vi "MIMIC RecvCommand_safe.vi"(3 "error in":errorcluster, 5 "VISA resource name":refnum<visa-resource-name>) -> (0 "error out":errorcluster, 1 "Receive_buffer":u8[](array[numeric]), 2 "VISA resource name OUT":refnum<visa-resource-name>)   [LabVIEW 2014]
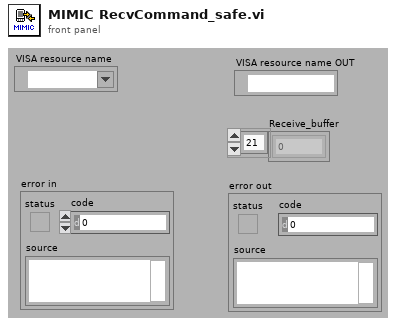
[diagram p1: front panel]
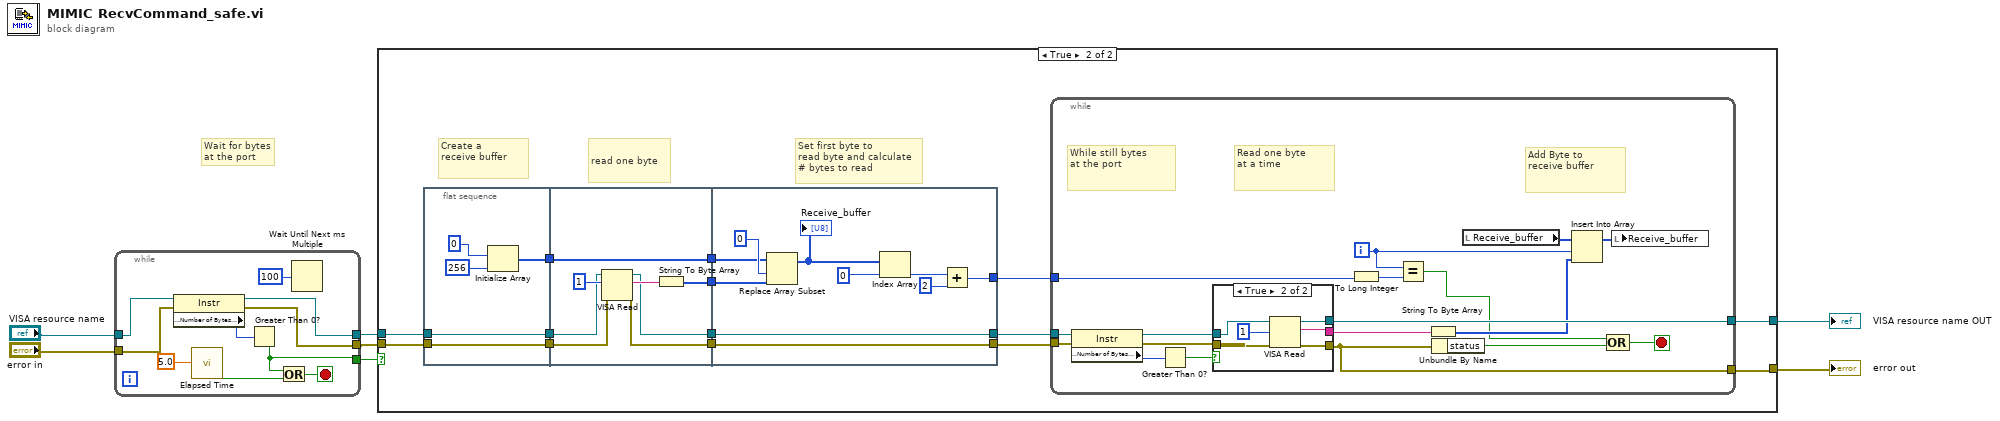
[diagram p0: block diagram]
diagram:
  # "Wait for bytes\nat the port"
  n1 = while {
    tunnel: "error in" -> [w10]
    tunnel: [w14] -> w7
    tunnel: "VISA resource name" -> [w13]
    tunnel: [w12] -> w6
    tunnel: [w8] -> w3
    stop <- w15 stop-if-true
    n2 = property class="Instr"(reference=w13, error in=w10) -> (reference out=w12:refnum<visa-resource-name>, error out=w14:errorcluster, "Serial Settings:Number of Bytes at Serial Port"=w17:u32)
    n3 = call "Elapsed Time"("Time Target (s)"=5.0) -> ("Time has Elapsed"=w16:bool)  [unwired: 11 in, 7 out]
    n4 = Greater Than 0?(x=w17) -> (x > 0?=w8:bool)
    n5 = Or(x=w8, y=w16) -> (x .or. y?=w15:bool)
    n6 = Wait Until Next ms Multiple(millisecond multiple=u32 100) -> ()  [unwired: 1 out]
  }
  n7 = case shown="True" w3 {
    tunnel: w7 -> [w18 w21]
    tunnel: w6 -> [w19 w22]
    tunnel: [w19 w33] -> w1
    tunnel: [w18 w32] -> w2
    frame False {
      # "No Bytes at the port, and we timed out"
    }
    frame True {
      # "Set first byte to \nread byte and calculate # bytes to read"
      # "read one byte"
      # "Create a\nreceive buffer"
      n8 = flat-sequence {
        tunnel: w22 -> [w37]
        tunnel: w21 -> [w38]
        tunnel: [w34] -> w25
        tunnel: [w38] -> w24
        tunnel: [w37] -> w23
        tunnel: [w39] -> w30
        tunnel: [w40] -> w29
        tunnel: [w42] -> w27
        tunnel: w25 -> [w39]
        tunnel: w24 -> [w41]
        tunnel: w23 -> [w43]
        tunnel: [w44] -> w20
        tunnel: [w52] -> w31
        tunnel: w30 -> [w47]
        tunnel: w29 -> [w50]
        tunnel: [w50] -> w28
        tunnel: w27 -> [w49]
        tunnel: [w49] -> w26
        tunnel: w20 -> [w48]
        frame #0 {
          n9 = Initialize Array(u8 0 ("element"), 256 ("dimension size")) -> (w34:u8[])
        }
        frame #1 {
          n10 = VISA Read(VISA resource name=w43, byte count=u32 1, error in (no error)=w41) -> (VISA resource name out=w42:refnum<visa-resource-name>, read buffer=w46:string, error out=w40:errorcluster)  [unwired: 1 out]
          n11 = String To Byte Array(string=w46) -> (unsigned byte array=w44:u8[])
        }
        frame #2 {
          n12 = Replace Array Subset(array=w47, new element=w48, index=0) -> (w56:u8[])
          "Receive_buffer" <- w56
          n13 = Index Array(array=w56, index=0) -> (element=w55:u8)
          n14 = Add(x=w55, y=u8 2) -> (x+y=w52:u8)
        }
      }
      n15 = while {
        tunnel: w26 -> [w72]
        tunnel: w28 -> [w71]
        tunnel: [w67] -> w33
        tunnel: [w64] -> w32
        tunnel: w31 -> [w61]
        i -> [w57]
        stop <- w68 stop-if-true
        # "Add Byte to \nreceive buffer"
        # "Read one byte\nat a time"
        # "While still bytes\nat the port"
        n16 = property class="Instr"(reference=w72, error in=w71) -> (reference out=w70:refnum<visa-resource-name>, error out=w69:errorcluster, "Serial Settings:Number of Bytes at Serial Port"=w74:u32)
        n17 = Greater Than 0?(x=w74) -> (x > 0?=w73:bool)
        n18 = case shown="True" w73 {
          tunnel: w69 -> [w76 w82]
          tunnel: w70 -> [w75 w81]
          tunnel: [w76 w80] -> w64
          tunnel: [_ w79] -> w66
          tunnel: [w75 w78] -> w67
          frame False {
          }
          frame True {
            n19 = VISA Read(VISA resource name=w81, byte count=u32 1, error in (no error)=w82) -> (VISA resource name out=w78:refnum<visa-resource-name>, read buffer=w79:string, error out=w80:errorcluster)  [unwired: 1 out]
          }
        }
        n20 = To Long Integer(number=w61) -> (32bit integer=w58:i32)
        n21 = Equal?(x=w57, y=w58) -> (x = y?=w60:bool)
        n22 = String To Byte Array(string=w66) -> (unsigned byte array=w65:u8[])
        n23 = Unbundle By Name(w64) -> ("status"=w59:bool)
        n24 = local read "Receive_buffer"() -> (w63:u8[])
        n25 = Insert Into Array(array=w63, index=w57, new element=w65) -> (w62:u8[])
        n26 = Compound Arithmetic op=OR(w60, w59) -> (w68:bool)
        n27 = local write "Receive_buffer"(w62) -> ()
      }
    }
  }
  "error out" <- w2
  "VISA resource name OUT" <- w1
